vi "Close.vi"(8 "error in (no error)":errorcluster, 11 "Pressure Control in":refnum<class "Pressure Control.lvclass">) -> (0 "error out":errorcluster, 3 "Pressure Control out":refnum<class "Pressure Control.lvclass">)   [LabVIEW 2011, in "Pressure Control.lvclass"]
uses:
  Pressure Control.lvclass
  Pressure Control.lvclass/Pressure Control.ctl
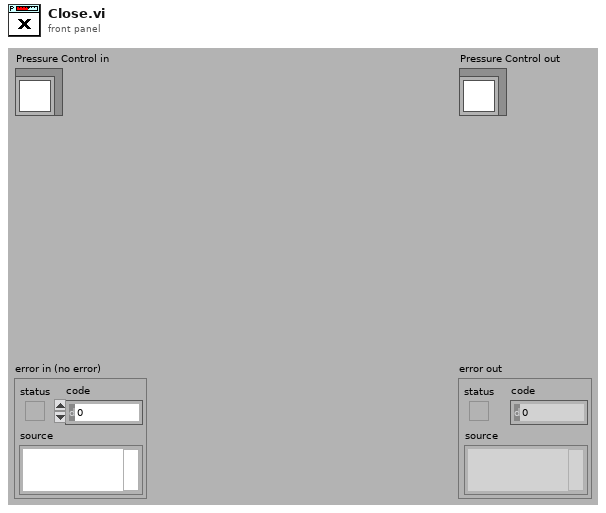
[diagram p1: front panel]
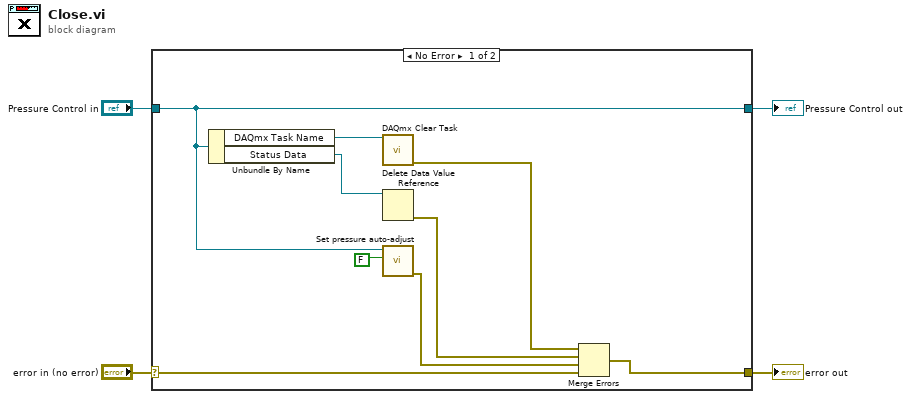
[diagram p0: block diagram]
diagram:
  n1 = case shown="No Error" "error in (no error)" {
    selector: "error in (no error)" -> [w11 w15]
    tunnel: [w10 w15] -> w3
    tunnel: [w7 w14] -> w1
    tunnel: "Pressure Control in" -> [w7 w14]
    frame No Error {
      n2 = Unbundle By Name(w7) -> ("DAQmx Task Name"=w13:refnum<k21>, "Status Data"=w12:refnum<data-value>)
      n3 = call <vilib>:"DAQmx Clear Task.vi"("task in"=w13) -> ("error out"=w9:errorcluster)  [unwired: 14 in]
      n4 = Delete Data Value Reference(data value reference=w12) -> (error out=w8:errorcluster)  [unwired: 1 in, 1 out]
      n5 = call "Set pressure auto-adjust.vi"("Enable?"=FALSE, "Pressure Control in"=w7) -> ("error out"=w5:errorcluster)  [unwired: 8 in, 1 out]
      n6 = Merge Errors(w9, w8, w5, w11) -> (w10:errorcluster)
    }
    frame Error {
    }
  }
  "error out" <- w3
  "Pressure Control out" <- w1
